vi "PathPlanner_PathFinding_SetDynamicObstacles.vi"(9 "CurrentRobotPosition":T1 {"Y" format="%14.3f"; "X" format="%14.3f"}, 11 "RectangularObstacles":T2[](array[typedef]) {"CornerPos2"."Y" format="%14.3f"; "CornerPos2"."X" format="%14.3f"; "CornerPos1"."Y" format="%14.3f"; "CornerPos1"."X" format="%14.3f"}) -> ()   [LabVIEW 2019, in "PathPlanner24.lvlib"]
uses:
  PathPlanner24.lvlib
  TypeDef/PathPlannerRectangularObstacle.ctl
  <vilib>/Rock Robotics/WPI/ThirdParty/JAS_Junk/TrajLib/TypeDef/TRANSLATION2D.ctl
  TypeDef/PathPlannerFinderGridPosition.ctl
  ENum/PathPlanner_PathFinding_Cmd_ENUM.ctl
  fc9fa233-4feb-4388-8dd1-d95799b98433.vi
  <vilib>/Rock Robotics/WPI/ThirdParty/JAS_Junk/TrajLib/Translation2d_GetXY.vi
  PathPlanner_PathFinder_Globals.vi
  <vilib>/Rock Robotics/WPI/ThirdParty/JAS_Junk/TrajLib/Trajectory_Library.lvlib
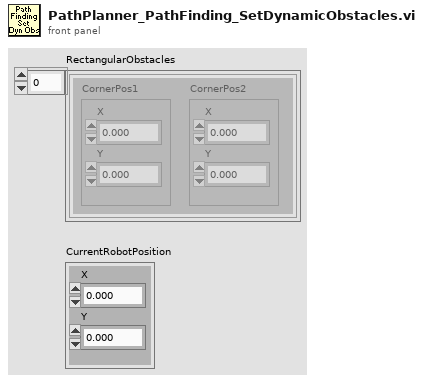
[diagram p1: front panel]
types:
  T1 = typedef "Trajectory_Library.lvlib/TRANSLATION2D.ctl" = cluster{"X":dbl, "Y":dbl}
  T2 = typedef "PathPlanner24.lvlib/PathPlannerRectangularObstacle.ctl" = cluster{"CornerPos1":T1, "CornerPos2":T1}
  T3 = typedef "PathPlanner24.lvlib/PathPlanner_PathFinding_Cmd_ENUM.ctl" = enum16{"Do Nothing", "Reset", "Minor", "Reset and Minor", "Major", "Reset and Major", "Minor and Major", "Reset, Minor, Major"}
  T4 = typedef "PathPlanner24.lvlib/PathPlannerFinderGridPosition.ctl" = cluster{"X":i32, "Y":i32}
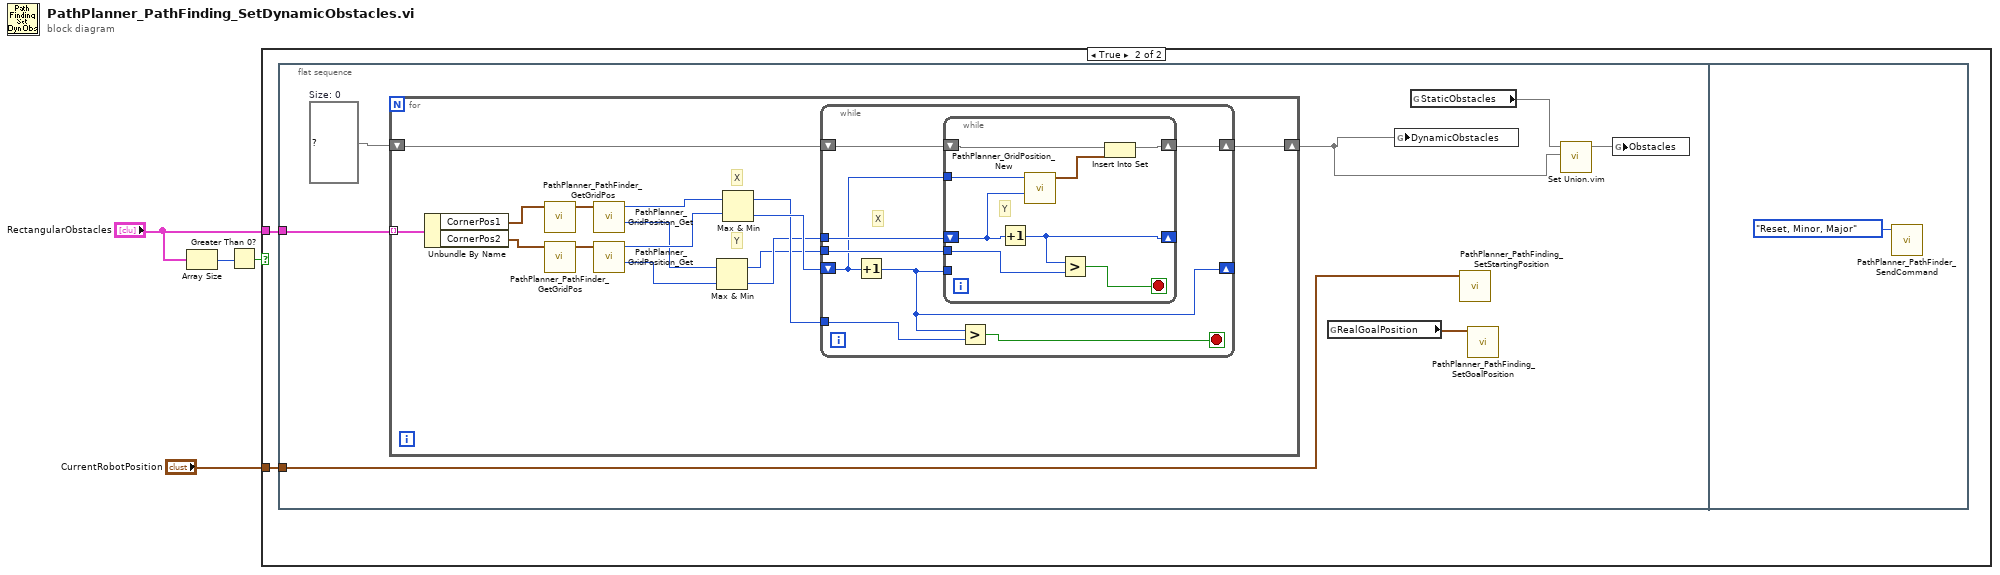
[diagram p0: block diagram]
diagram:
  n1 = Array Size(array="RectangularObstacles") -> (size(s)=w4:i32)
  n2 = Greater Than 0?(x=w4) -> (x > 0?=w3:bool)
  n3 = case shown="True" w3 {
    tunnel: "RectangularObstacles" -> [_ w6]
    tunnel: "CurrentRobotPosition" -> [_ w5]
    frame False {
    }
    frame True {
      n4 = flat-sequence {
        tunnel: w6 -> [w13]
        tunnel: w5 -> [w11]
        frame #0 {
          w10 = set{T4} {}  # Size: 0
          n5 = for {
            tunnel: w13 -> [w28] mode=indexing
            shift-right: [w14] -> w8
            shift-left: w10 -> [w23]
            # "Y"
            # "X"
            n6 = Unbundle By Name(w28) -> ("CornerPos1"=w22:T1, "CornerPos2"=w21:T1)
            n7 = call "PathPlanner_PathFinder_GetGridPos.vi"("RealGridPos"=w22) -> ("GridPosition"=w20:T4)  [unwired: 10 in]
            n8 = call "PathPlanner_PathFinder_GetGridPos.vi"("RealGridPos"=w21) -> ("GridPosition"=w19:T4)  [unwired: 10 in]
            n9 = call "PathPlanner_GridPosition_Get.vi"("GridPosition"=w20) -> ("Y"=w16:i32, "X"=w18:i32)  [unwired: 9 in]
            n10 = call "PathPlanner_GridPosition_Get.vi"("GridPosition"=w19) -> ("Y"=w15:i32, "X"=w17:i32)  [unwired: 9 in]
            n11 = Max & Min(x=w16, y=w15) -> (max(x,y)=w24:i32, min(x,y)=w25:i32)
            n12 = Max & Min(x=w18, y=w17) -> (max(x,y)=w26:i32, min(x,y)=w27:i32)
            n13 = while {
              shift-right: [w33] -> _
              shift-left: w27 -> [w30]
              tunnel: w26 -> [w36]
              tunnel: w25 -> [w34]
              tunnel: w24 -> [w32]
              shift-right: [w29] -> w14
              shift-left: w23 -> [w31]
              stop <- w35 stop-if-true
              # "X"
              n14 = Increment(x=w30) -> (x+1=w33:i32)
              n15 = while {
                shift-right: [w44] -> _
                shift-left: w34 -> [w41]
                tunnel: w33 -> [_]
                tunnel: w32 -> [w43]
                shift-right: [w39] -> w29
                shift-left: w31 -> [w38]
                tunnel: w30 -> [w40]
                stop <- w42 stop-if-true
                # "Y"
                n16 = Increment(x=w41) -> (x+1=w44:i32)
                n17 = call "PathPlanner_GridPosition_New.vi"("Y"=w41, "X"=w40) -> ("GridPosition"=w37:T4)  [unwired: 9 in]
                n18 = Greater?(x=w44, y=w43) -> (0:w42:bool)
                n19 = Insert Into Set(10:w37, 11:w38) -> (3:w39:set{T4})  [unwired: 1 out]
              }
              n20 = Greater?(x=w33, y=w36) -> (0:w35:bool)
            }
          }
          n21 = global read "PathPlanner_PathFinder_Globals.vi" "RealGoalPosition"() -> (w12:T1)
          n22 = global write "PathPlanner_PathFinder_Globals.vi" "DynamicObstacles"(w8) -> ()
          n23 = global read "PathPlanner_PathFinder_Globals.vi" "StaticObstacles"() -> (w9:set{T4})
          n24 = call "PathPlanner_PathFinding_SetStartingPosition.vi"("StartPosition"=w11) -> ()  [unwired: 11 in]
          n25 = call "PathPlanner_PathFinding_SetGoalPosition.vi"("GoalPosition"=w12) -> ()  [unwired: 11 in]
          n26 = call "Set Union.vim"("set 2"=w8, "set 1"=w9) -> ("union"=w7:set{T4})  [unwired: 9 in]
          n27 = global write "PathPlanner_PathFinder_Globals.vi" "Obstacles"(w7) -> ()
        }
        frame #1 {
          n28 = call "PathPlanner_PathFinder_SendCommand.vi"("PathFindingCommand"=PathPlanner_PathFinding_Cmd_ENUM."Reset, Minor, Major") -> ()  [unwired: 10 in, 1 out]
        }
      }
    }
  }
